vi "Identify.vi"(8 "error in (no error)":errorcluster, 11 "SPECAN_PVT in":refnum<class "SPECAN_PVT.lvclass">) -> (0 "error out":errorcluster, 2 "Plugin is Valid":bool, 3 "SPECAN_PVT out":refnum<class "SPECAN_PVT.lvclass">)   [LabVIEW 2018, in "SPECAN_PVT.lvlib" / "SPECAN_PVT.lvclass"]
uses:
  SPECAN_PVT.lvclass
  C:/Sequence Automation/Plugins/Measurement Interface.lvlibp/Measurement Interface.lvclass
  Plugins/Measurement Interface.lvlibp/Private Methods/Measurement Definition Entry/Read Measurement Definition Entry.vi
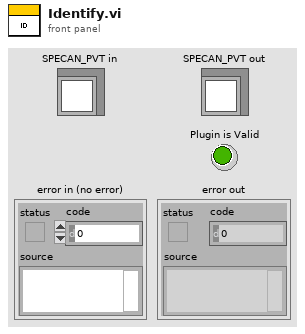
[diagram p1: front panel]
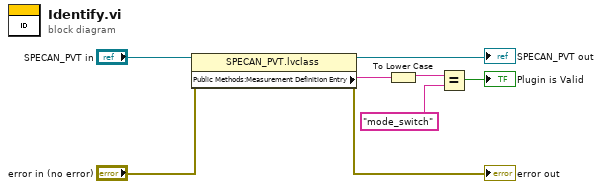
[diagram p0: block diagram]
diagram:
  n1 = property class="SPECAN_PVT.lvclass"(reference="SPECAN_PVT in", error in="error in (no error)") -> (reference out=→"SPECAN_PVT out":refnum<class "SPECAN_PVT.lvclass">, error out=→"error out":errorcluster, "Public Methods:Measurement Definition Entry"=w7:string)
  n2 = To Lower Case(string=w7) -> (all lower case string=w5:string)
  n3 = Equal?(x=w5, y="mode_switch") -> (x = y?=→"Plugin is Valid":bool)
